vi "main.vi"() -> ()   [LabVIEW 2024]
uses:
  Controls/#typedef_program_data.ctl
  Controls/#typedef_steps.ctl
  Controls/#typedef_program_states_kawa.ctl
  Controls/#typedef_action_timer.ctl
panel:
  out "error out":errorcluster
  in  "error in (no error)":errorcluster
  in  "Cluster":T1
  in  "stop":bool
  out "Whipped Cream":bool
  out "Chocolate Syrup":bool
  out "Milk Foam":bool
  out "Steamed Milk":bool
  out "Espresso":bool
  in  "Cafe Mocha":bool
  in  "Cafe Latte":bool
  in  "Espresso Macchiato":bool
  in  "Espresso":bool
  # "Wybierz kawe:"
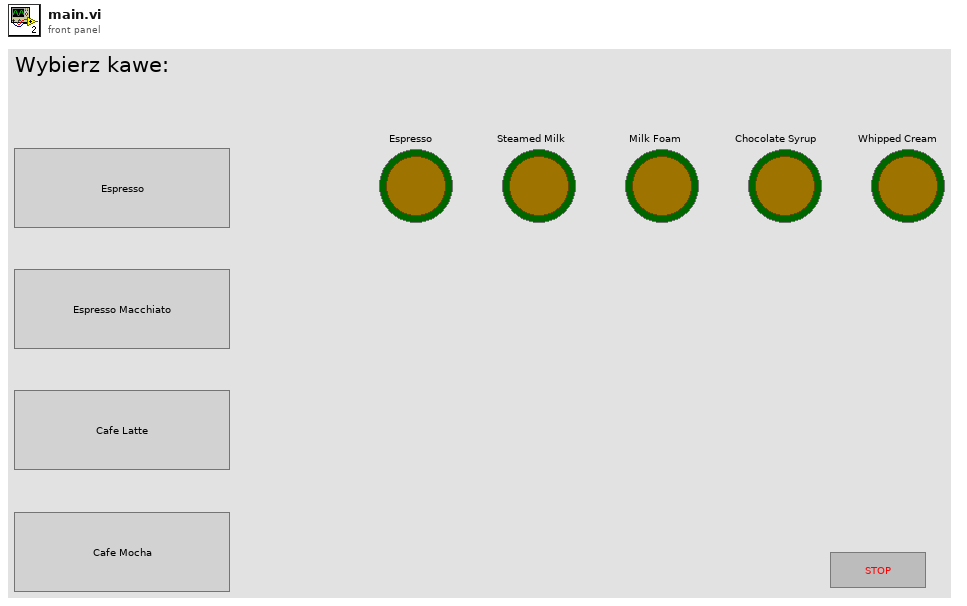
[diagram p1: front panel]
types:
  T1 = typedef "#typedef_program_data.ctl" = cluster{"Espresso":bool, "Steamed Milk":bool, "Milk Foam":bool, "Chocolate Syrup":bool, "Whipped Cream":bool, "steps":T2}
  T2 = typedef "#typedef_steps.ctl" = enum16{"start", "espresso", "chocolate syrup", "steamed milk", "milk foam", "whipped cream", "end"}
  T3 = typedef "#typedef_program_states_kawa.ctl" = enum16{"Application Error", "init", "idle", "espresso", "espresso macchiato", "caffe latte", "cafe mocha", "stop"}
  T4 = enum8{"Enabled", "Disabled", "Disabled and Grayed Out"}
  T5 = typedef "#typedef_action_timer.ctl" = enum16{"reset", "timeElapsed"}
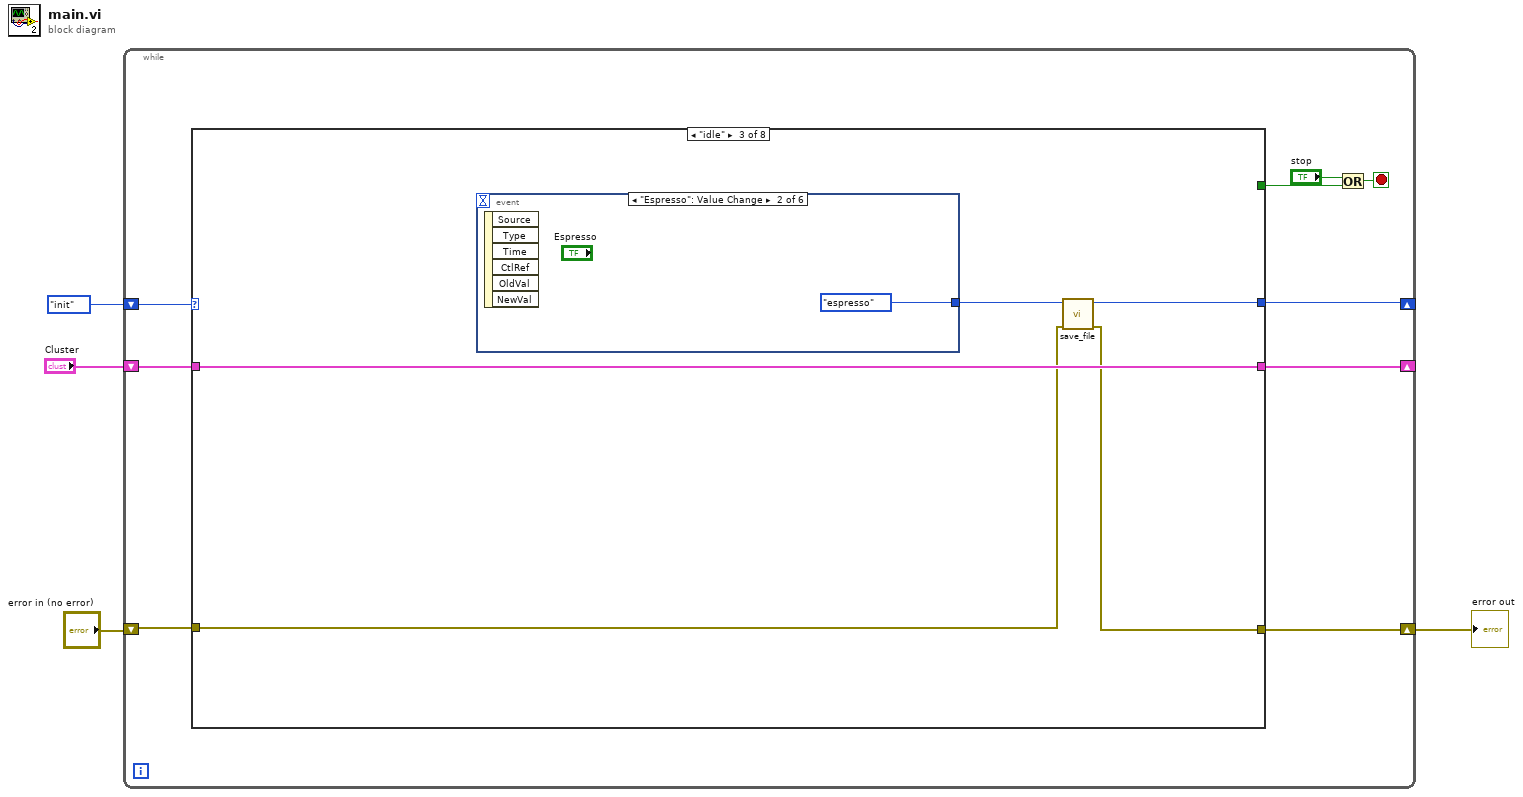
[diagram p0: block diagram]
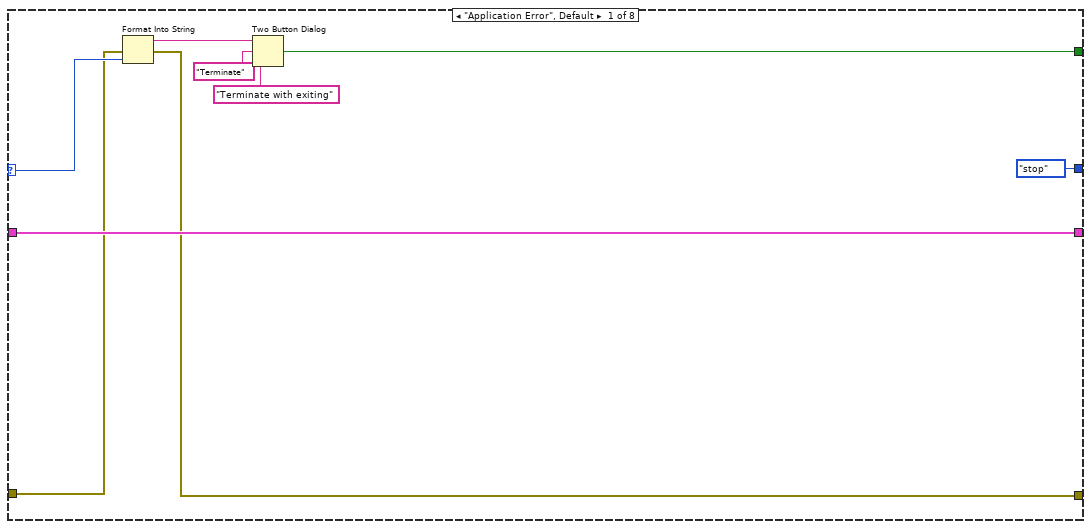
[diagram p2: hidden frame]
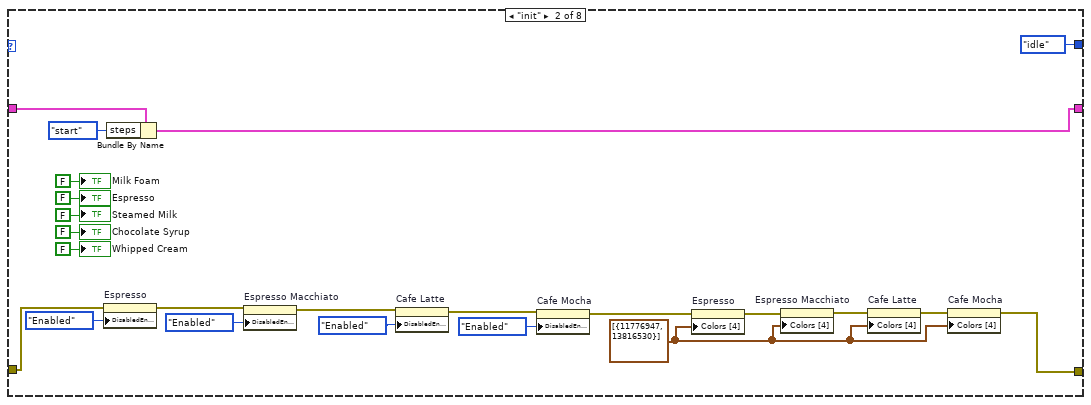
[diagram p3: hidden frame]
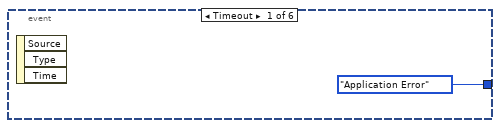
[diagram p4: hidden frame]
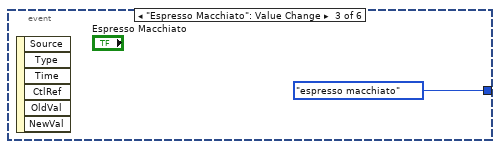
[diagram p5: hidden frame]
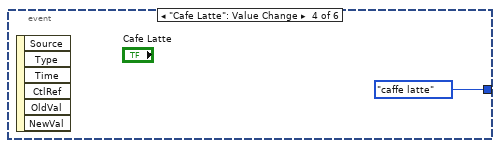
[diagram p6: hidden frame]
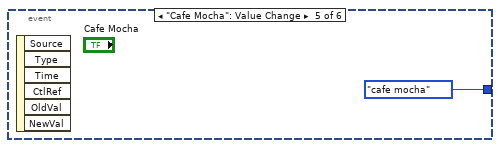
[diagram p7: hidden frame]
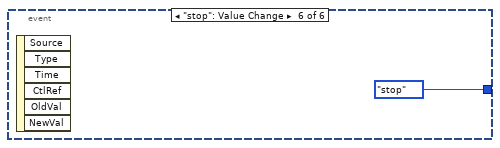
[diagram p8: hidden frame]
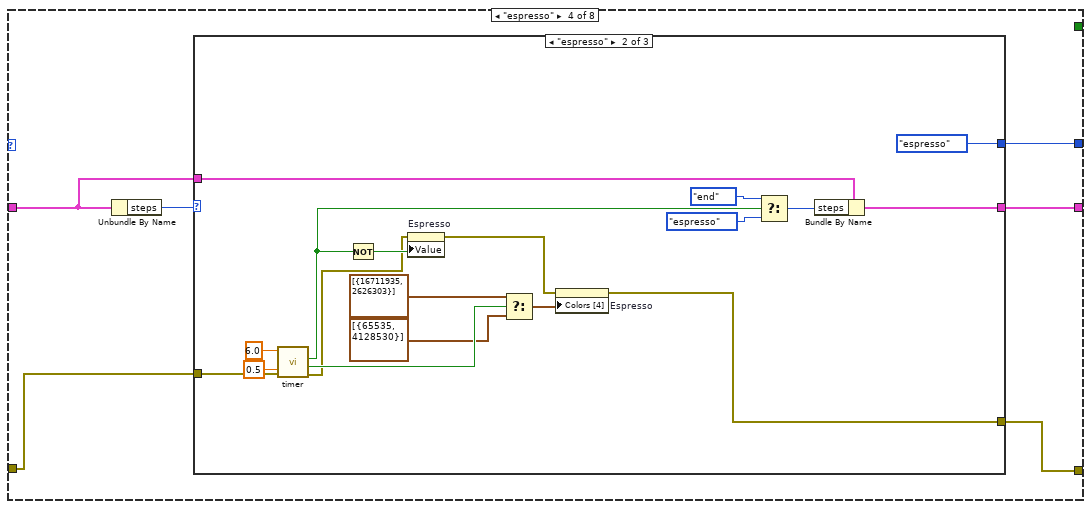
[diagram p9: hidden frame]
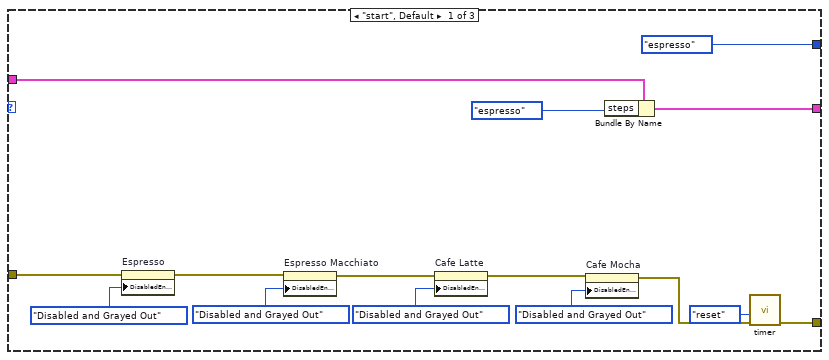
[diagram p10: hidden frame]
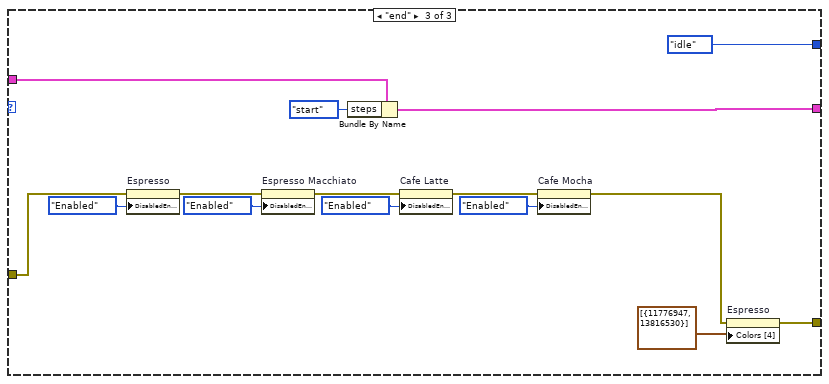
[diagram p11: hidden frame]
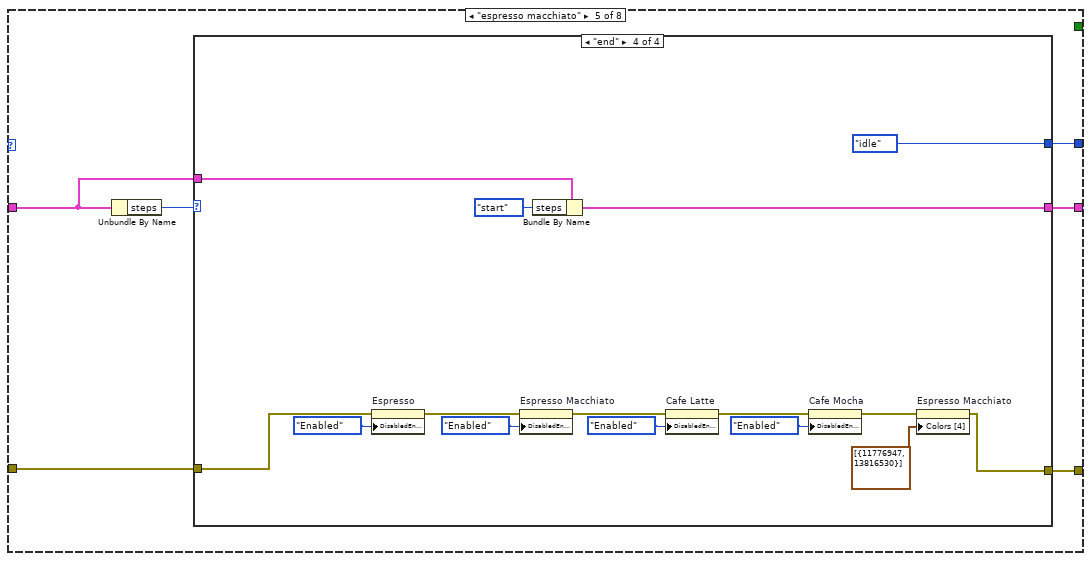
[diagram p12: hidden frame]
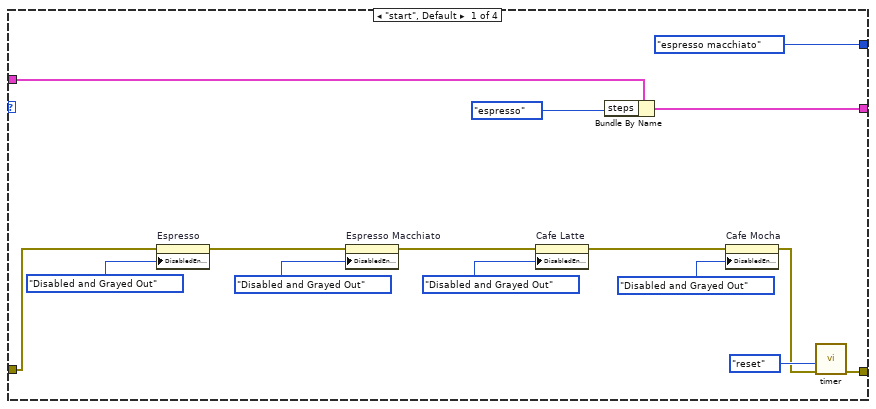
[diagram p13: hidden frame]
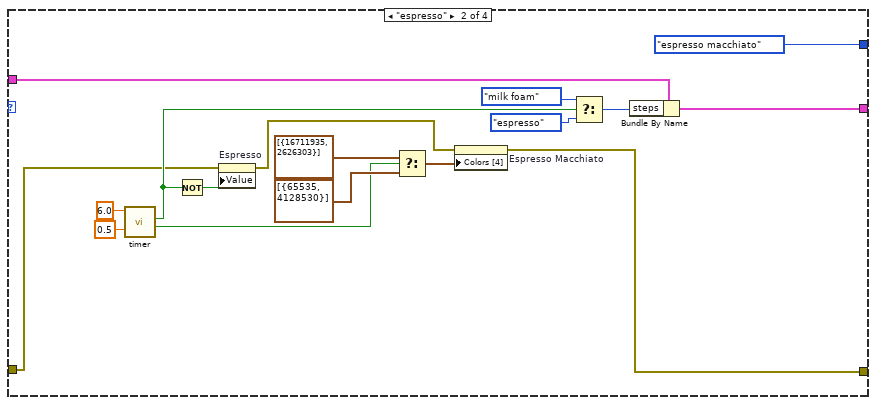
[diagram p14: hidden frame]
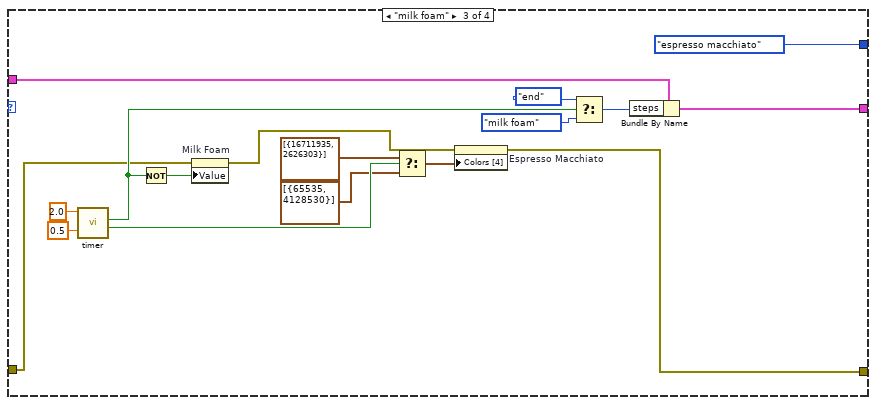
[diagram p15: hidden frame]
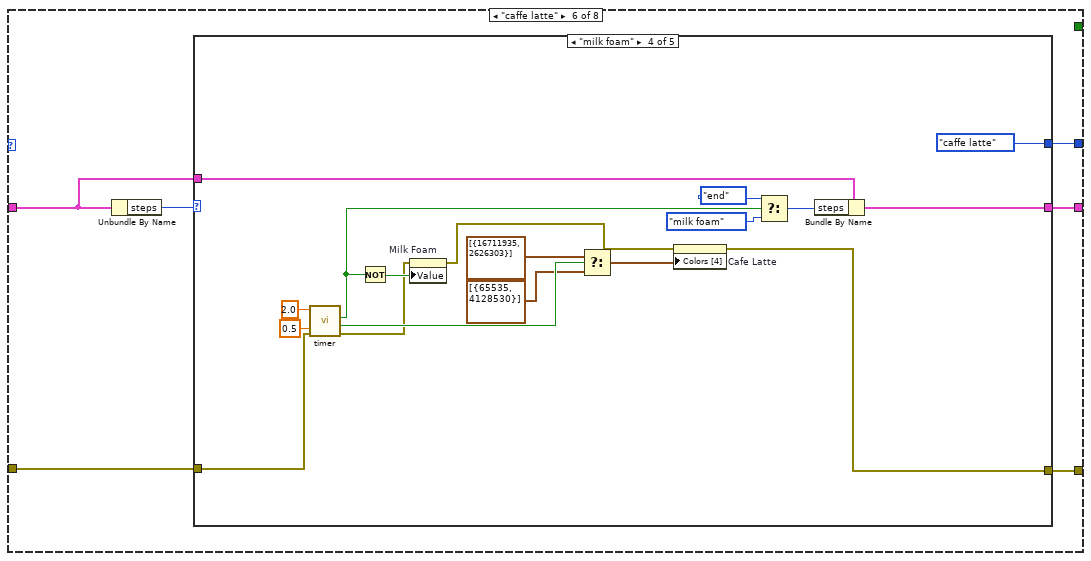
[diagram p16: hidden frame]
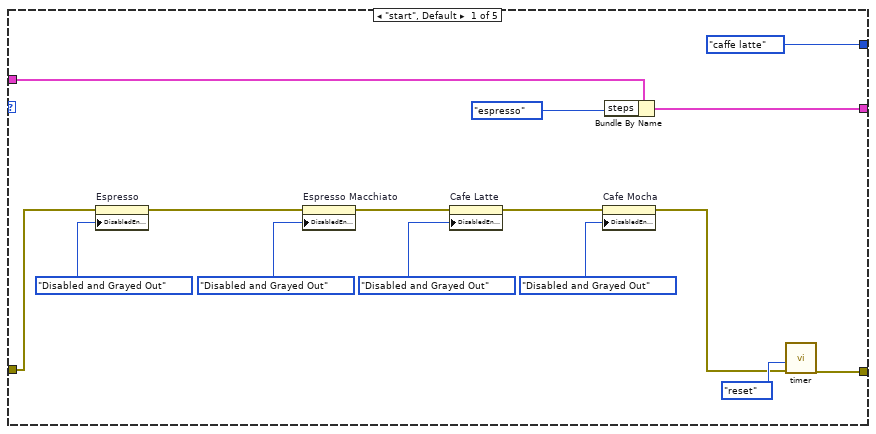
[diagram p17: hidden frame]
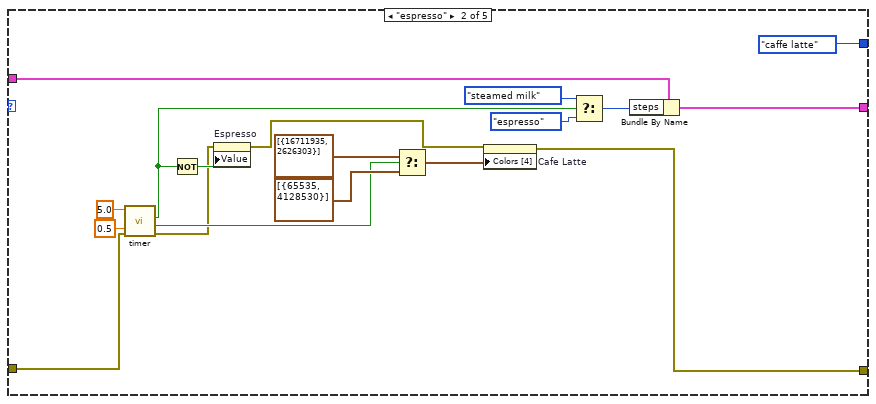
[diagram p18: hidden frame]
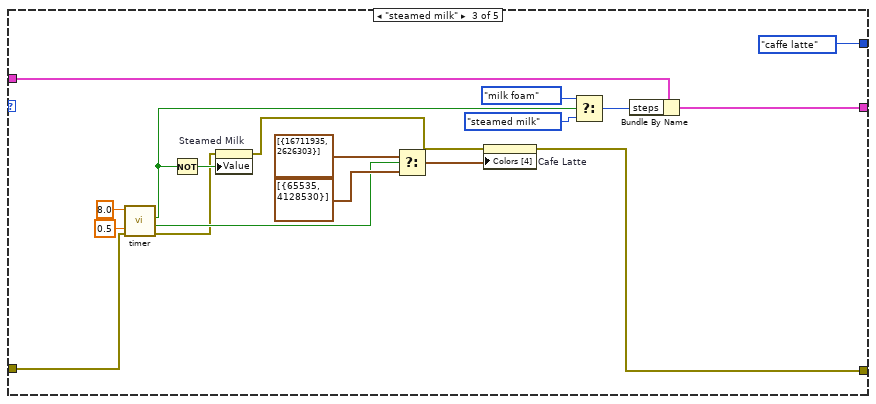
[diagram p19: hidden frame]
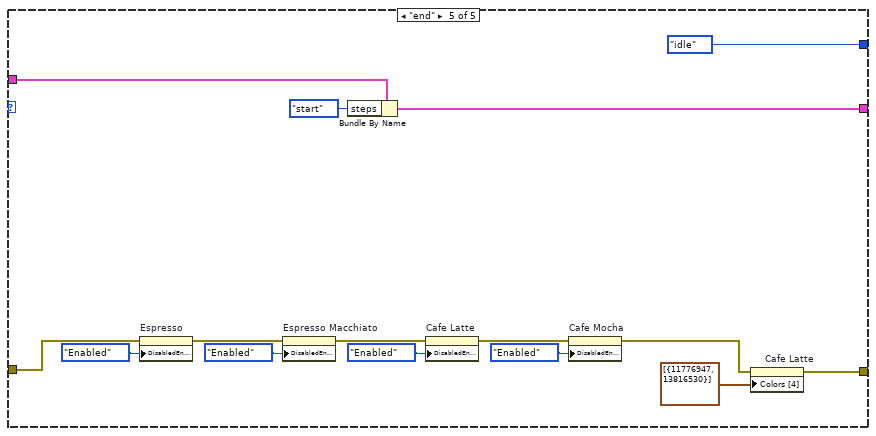
[diagram p20: hidden frame]
diagram:
  n1 = while {
    shift-right: [w11] -> _
    shift-left: #typedef_program_states_kawa."init" ("program states") -> [w13]
    shift-right: [w9] -> _
    shift-left: "Cluster" -> [w10]
    shift-right: [w5] -> w1
    shift-left: "error in (no error)" -> [w6]
    stop <- w8 stop-if-true
    n2 = case shown="\"idle\"" w13 {
      selector: w13 -> [w21 _ _ _ _ _ _ _]
      tunnel: [w17 _ _ _ _ _ _ TRUE ("T button?")] -> w12
      tunnel: [#typedef_program_states_kawa."stop" ("program states") #typedef_program_states_kawa."idle" ("program states") w48 w59 w113 w183 w273 #typedef_program_states_kawa."Application Error" ("program states")] -> w11
      tunnel: w10 -> [w16 w39 w50 w61 w115 w185 w275 w381]
      tunnel: [w16 w37 w50 w60 w114 w184 w274 w381] -> w9
      tunnel: w6 -> [w15 w31 w47 w58 w112 w182 w272 w379]
      tunnel: [w14 w23 w46 w57 w111 w181 w271 w379] -> w5
      frame "Application Error", Default {
        n3 = Format Into String(error in=w15, w21) -> (resulting string=w20:string, error out=w14:errorcluster)  [unwired: 2 in]
        n4 = Two Button Dialog(message=w20, 1:"Terminate with exiting" ("F button name (\"Cancel\")"), 2:"Terminate" ("T button name (\"OK\")")) -> (T button?=w17:bool)
      }
      frame "init" {
        w32 = cluster{u32, u32}[] [{11776947, 13816530}] ("Colors [4]")
        n5 = property on="Espresso" class="Bool"(error in=w31, "DisabledEnum"=T4."Enabled" ("Disabled")) -> (error out=w30:errorcluster)  [unwired: 1 in, 1 out]
        n6 = Bundle By Name(cluster=w39, "steps"=#typedef_steps."start") -> (w37:T1)
        n7 = property on="Espresso Macchiato" class="Bool"(error in=w30, "DisabledEnum"=T4."Enabled" ("Disabled")) -> (error out=w29:errorcluster)  [unwired: 1 in, 1 out]
        n8 = property on="Cafe Latte" class="Bool"(error in=w29, "DisabledEnum"=T4."Enabled" ("Disabled")) -> (error out=w28:errorcluster)  [unwired: 1 in, 1 out]
        n9 = property on="Cafe Mocha" class="Bool"(error in=w28, "DisabledEnum"=T4."Enabled" ("Disabled")) -> (error out=w27:errorcluster)  [unwired: 1 in, 1 out]
        n10 = property on="Espresso" class="Bool"(error in=w27, "Colors [4]"=w32) -> (error out=w26:errorcluster)  [unwired: 1 in, 1 out]
        n11 = property on="Espresso Macchiato" class="Bool"(error in=w26, "Colors [4]"=w32) -> (error out=w25:errorcluster)  [unwired: 1 in, 1 out]
        n12 = property on="Cafe Latte" class="Bool"(error in=w25, "Colors [4]"=w32) -> (error out=w24:errorcluster)  [unwired: 1 in, 1 out]
        n13 = property on="Cafe Mocha" class="Bool"(error in=w24, "Colors [4]"=w32) -> (error out=w23:errorcluster)  [unwired: 1 in, 1 out]
        "Espresso" <- FALSE ("Milk Foam")
        "Steamed Milk" <- FALSE ("Milk Foam")
        "Milk Foam" <- FALSE ("Milk Foam")
        "Chocolate Syrup" <- FALSE ("Milk Foam")
        "Whipped Cream" <- FALSE ("Milk Foam")
      }
      frame "idle" {
        n14 = event shown="[1] \"Espresso\": Value Change" {
          selector: _ -> [_ _ _ _ _ _]
          dyn-events: _ -> [_ _ _ _ _ _]
          timeout: _ -> [_ _ _ _ _ _]
          tunnel: [#typedef_program_states_kawa."Application Error" ("program states") #typedef_program_states_kawa."espresso" ("program states") #typedef_program_states_kawa."espresso macchiato" ("program states") #typedef_program_states_kawa."caffe latte" ("program states") #typedef_program_states_kawa."cafe mocha" ("program states") #typedef_program_states_kawa."stop" ("program states")] -> w49
          event Timeout {
            n15 = event-data() -> ()  [unwired: 1 in, 3 out]
          }
          event "Espresso": Value Change {
            n16 = event-data() -> ()  [unwired: 1 in, 6 out]
          }
          event "Espresso Macchiato": Value Change {
            n17 = event-data() -> ()  [unwired: 1 in, 6 out]
          }
          event "Cafe Latte": Value Change {
            n18 = event-data() -> ()  [unwired: 1 in, 6 out]
          }
          event "Cafe Mocha": Value Change {
            n19 = event-data() -> ()  [unwired: 1 in, 6 out]
          }
          event "stop": Value Change {
            n20 = event-data() -> ()  [unwired: 1 in, 6 out]
          }
        }
        n21 = call "save_file.vi"("error in (no error)"=w47, "program states  in"=w49) -> ("error out"=w46:errorcluster, "program states out"=w48:T3)  [unwired: 8 in]
      }
      frame "espresso" {
        n22 = Unbundle By Name(w61) -> ("steps"=w62:T2)
        n23 = case shown="\"espresso\"" w62 {
          tunnel: w61 -> [w77 w91 w109]
          tunnel: [w75 w92 w108] -> w60
          tunnel: [#typedef_program_states_kawa."espresso" ("program states") #typedef_program_states_kawa."espresso" ("program states") #typedef_program_states_kawa."idle" ("program states")] -> w59
          tunnel: w58 -> [w68 w81 w96]
          tunnel: [w63 w78 w101] -> w57
          frame "start", Default {
            n24 = property on="Espresso" class="Bool"(error in=w68, "DisabledEnum"=T4."Disabled and Grayed Out" ("Disabled")) -> (error out=w67:errorcluster)  [unwired: 1 in, 1 out]
            n25 = property on="Espresso Macchiato" class="Bool"(error in=w67, "DisabledEnum"=T4."Disabled and Grayed Out" ("Disabled")) -> (error out=w66:errorcluster)  [unwired: 1 in, 1 out]
            n26 = property on="Cafe Latte" class="Bool"(error in=w66, "DisabledEnum"=T4."Disabled and Grayed Out" ("Disabled")) -> (error out=w65:errorcluster)  [unwired: 1 in, 1 out]
            n27 = property on="Cafe Mocha" class="Bool"(error in=w65, "DisabledEnum"=T4."Disabled and Grayed Out" ("Disabled")) -> (error out=w64:errorcluster)  [unwired: 1 in, 1 out]
            n28 = Bundle By Name(cluster=w77, "steps"=#typedef_steps."espresso") -> (w75:T1)
            n29 = call "timer.vi"("error in (no error)"=w64, "action"=#typedef_action_timer."reset") -> ("error out"=w63:errorcluster)  [unwired: 6 in, 3 out]
          }
          frame "espresso" {
            n30 = call "timer.vi"("error in (no error)"=w81, "Time to elapse latch"=0.5, "Time to elapse (s)"=6.0) -> ("error out"=w80:errorcluster, "time elapsed latch"=w84:bool, "timeElapsed?"=w93:bool)  [unwired: 5 in, 1 out]
            n31 = Not(x=w93) -> (.not. x?=w95:bool)
            n32 = property on="Espresso" class="Bool (strict)"(error in=w80, "Value"=w95) -> (error out=w79:errorcluster)  [unwired: 1 in, 1 out]
            n33 = Select(t=cluster{u32, u32}[] [{16711935, 2626303}] ("Colors [4]"), s=w84, f=cluster{u32, u32}[] [{65535, 4128530}] ("Colors [4]")) -> (s? t:f=w86:cluster{u32, u32}[])
            n34 = property on="Espresso" class="Bool"(error in=w79, "Colors [4]"=w86) -> (error out=w78:errorcluster)  [unwired: 1 in, 1 out]
            n35 = Select(t=#typedef_steps."end" ("steps"), s=w93, f=#typedef_steps."espresso" ("steps")) -> (s? t:f=w88:T2)
            n36 = Bundle By Name(cluster=w91, "steps"=w88) -> (w92:T1)
          }
          frame "end" {
            n37 = property on="Espresso" class="Bool"(error in=w96, "DisabledEnum"=T4."Enabled" ("Disabled")) -> (error out=w97:errorcluster)  [unwired: 1 in, 1 out]
            n38 = property on="Espresso Macchiato" class="Bool"(error in=w97, "DisabledEnum"=T4."Enabled" ("Disabled")) -> (error out=w98:errorcluster)  [unwired: 1 in, 1 out]
            n39 = Bundle By Name(cluster=w109, "steps"=#typedef_steps."start") -> (w108:T1)
            n40 = property on="Cafe Latte" class="Bool"(error in=w98, "DisabledEnum"=T4."Enabled" ("Disabled")) -> (error out=w99:errorcluster)  [unwired: 1 in, 1 out]
            n41 = property on="Cafe Mocha" class="Bool"(error in=w99, "DisabledEnum"=T4."Enabled" ("Disabled")) -> (error out=w100:errorcluster)  [unwired: 1 in, 1 out]
            n42 = property on="Espresso" class="Bool"(error in=w100, "Colors [4]"=cluster{u32, u32}[] [{11776947, 13816530}]) -> (error out=w101:errorcluster)  [unwired: 1 in, 1 out]
          }
        }
      }
      frame "espresso macchiato" {
        n43 = Unbundle By Name(w115) -> ("steps"=w116:T2)
        n44 = case shown="\"end\"" w116 {
          tunnel: w115 -> [w131 w144 w162 w179]
          tunnel: [w129 w145 w163 w178] -> w114
          tunnel: [#typedef_program_states_kawa."espresso macchiato" ("program states") #typedef_program_states_kawa."espresso macchiato" ("program states") #typedef_program_states_kawa."espresso macchiato" ("program states") #typedef_program_states_kawa."idle" ("program states")] -> w113
          tunnel: w112 -> [w122 w134 w151 w171]
          tunnel: [w117 w132 w149 w166] -> w111
          frame "start", Default {
            n45 = property on="Espresso" class="Bool"(error in=w122, "DisabledEnum"=T4."Disabled and Grayed Out" ("Disabled")) -> (error out=w121:errorcluster)  [unwired: 1 in, 1 out]
            n46 = property on="Espresso Macchiato" class="Bool"(error in=w121, "DisabledEnum"=T4."Disabled and Grayed Out" ("Disabled")) -> (error out=w120:errorcluster)  [unwired: 1 in, 1 out]
            n47 = property on="Cafe Latte" class="Bool"(error in=w120, "DisabledEnum"=T4."Disabled and Grayed Out" ("Disabled")) -> (error out=w119:errorcluster)  [unwired: 1 in, 1 out]
            n48 = Bundle By Name(cluster=w131, "steps"=#typedef_steps."espresso") -> (w129:T1)
            n49 = property on="Cafe Mocha" class="Bool"(error in=w119, "DisabledEnum"=T4."Disabled and Grayed Out" ("Disabled")) -> (error out=w118:errorcluster)  [unwired: 1 in, 1 out]
            n50 = call "timer.vi"("error in (no error)"=w118, "action"=#typedef_action_timer."reset") -> ("error out"=w117:errorcluster)  [unwired: 6 in, 3 out]
          }
          frame "espresso" {
            n51 = call "timer.vi"("Time to elapse latch"=0.5, "Time to elapse (s)"=6.0) -> ("time elapsed latch"=w136:bool, "timeElapsed?"=w146:bool)  [unwired: 6 in, 2 out]
            n52 = Not(x=w146) -> (.not. x?=w148:bool)
            n53 = property on="Espresso" class="Bool (strict)"(error in=w134, "Value"=w148) -> (error out=w133:errorcluster)  [unwired: 1 in, 1 out]
            n54 = Select(t=cluster{u32, u32}[] [{16711935, 2626303}] ("Colors [4]"), s=w136, f=cluster{u32, u32}[] [{65535, 4128530}] ("Colors [4]")) -> (s? t:f=w135:cluster{u32, u32}[])
            n55 = property on="Espresso Macchiato" class="Bool"(error in=w133, "Colors [4]"=w135) -> (error out=w132:errorcluster)  [unwired: 1 in, 1 out]
            n56 = Select(t=#typedef_steps."milk foam" ("steps"), s=w146, f=#typedef_steps."espresso" ("steps")) -> (s? t:f=w141:T2)
            n57 = Bundle By Name(cluster=w144, "steps"=w141) -> (w145:T1)
          }
          frame "milk foam" {
            n58 = call "timer.vi"("Time to elapse latch"=0.5, "Time to elapse (s)"=2.0) -> ("time elapsed latch"=w156:bool, "timeElapsed?"=w164:bool)  [unwired: 6 in, 2 out]
            n59 = Not(x=w164) -> (.not. x?=w152:bool)
            n60 = property on="Milk Foam" class="Bool (strict)"(error in=w151, "Value"=w152) -> (error out=w150:errorcluster)  [unwired: 1 in, 1 out]
            n61 = Select(t=cluster{u32, u32}[] [{16711935, 2626303}] ("Colors [4]"), s=w156, f=cluster{u32, u32}[] [{65535, 4128530}] ("Colors [4]")) -> (s? t:f=w155:cluster{u32, u32}[])
            n62 = property on="Espresso Macchiato" class="Bool"(error in=w150, "Colors [4]"=w155) -> (error out=w149:errorcluster)  [unwired: 1 in, 1 out]
            n63 = Select(t=#typedef_steps."end" ("steps"), s=w164, f=#typedef_steps."milk foam" ("steps")) -> (s? t:f=w159:T2)
            n64 = Bundle By Name(cluster=w162, "steps"=w159) -> (w163:T1)
          }
          frame "end" {
            n65 = property on="Espresso" class="Bool"(error in=w171, "DisabledEnum"=T4."Enabled" ("Disabled")) -> (error out=w170:errorcluster)  [unwired: 1 in, 1 out]
            n66 = property on="Espresso Macchiato" class="Bool"(error in=w170, "DisabledEnum"=T4."Enabled" ("Disabled")) -> (error out=w169:errorcluster)  [unwired: 1 in, 1 out]
            n67 = Bundle By Name(cluster=w179, "steps"=#typedef_steps."start") -> (w178:T1)
            n68 = property on="Cafe Latte" class="Bool"(error in=w169, "DisabledEnum"=T4."Enabled" ("Disabled")) -> (error out=w168:errorcluster)  [unwired: 1 in, 1 out]
            n69 = property on="Cafe Mocha" class="Bool"(error in=w168, "DisabledEnum"=T4."Enabled" ("Disabled")) -> (error out=w167:errorcluster)  [unwired: 1 in, 1 out]
            n70 = property on="Espresso Macchiato" class="Bool"(error in=w167, "Colors [4]"=cluster{u32, u32}[] [{11776947, 13816530}]) -> (error out=w166:errorcluster)  [unwired: 1 in, 1 out]
          }
        }
      }
      frame "caffe latte" {
        n71 = Unbundle By Name(w185) -> ("steps"=w186:T2)
        n72 = case shown="\"milk foam\"" w186 {
          tunnel: w185 -> [w201 w215 w234 w252 w269]
          tunnel: [w199 w216 w235 w253 w268] -> w184
          tunnel: [#typedef_program_states_kawa."caffe latte" ("program states") #typedef_program_states_kawa."caffe latte" ("program states") #typedef_program_states_kawa."caffe latte" ("program states") #typedef_program_states_kawa."caffe latte" ("program states") #typedef_program_states_kawa."idle" ("program states")] -> w183
          tunnel: w182 -> [w187 w202 w220 w238 w261]
          tunnel: [w192 w204 w222 w240 w256] -> w181
          frame "start", Default {
            n73 = property on="Espresso" class="Bool"(error in=w187, "DisabledEnum"=T4."Disabled and Grayed Out" ("Disabled")) -> (error out=w188:errorcluster)  [unwired: 1 in, 1 out]
            n74 = property on="Espresso Macchiato" class="Bool"(error in=w188, "DisabledEnum"=T4."Disabled and Grayed Out" ("Disabled")) -> (error out=w189:errorcluster)  [unwired: 1 in, 1 out]
            n75 = property on="Cafe Latte" class="Bool"(error in=w189, "DisabledEnum"=T4."Disabled and Grayed Out" ("Disabled")) -> (error out=w190:errorcluster)  [unwired: 1 in, 1 out]
            n76 = property on="Cafe Mocha" class="Bool"(error in=w190, "DisabledEnum"=T4."Disabled and Grayed Out" ("Disabled")) -> (error out=w191:errorcluster)  [unwired: 1 in, 1 out]
            n77 = Bundle By Name(cluster=w201, "steps"=#typedef_steps."espresso") -> (w199:T1)
            n78 = call "timer.vi"("error in (no error)"=w191, "action"=#typedef_action_timer."reset") -> ("error out"=w192:errorcluster)  [unwired: 6 in, 3 out]
          }
          frame "espresso" {
            n79 = call "timer.vi"("error in (no error)"=w202, "Time to elapse latch"=0.5, "Time to elapse (s)"=5.0) -> ("error out"=w203:errorcluster, "time elapsed latch"=w207:bool, "timeElapsed?"=w217:bool)  [unwired: 5 in, 1 out]
            n80 = Not(x=w217) -> (.not. x?=w219:bool)
            n81 = property on="Espresso" class="Bool (strict)"(error in=w203, "Value"=w219) -> (error out=w205:errorcluster)  [unwired: 1 in, 1 out]
            n82 = Select(t=cluster{u32, u32}[] [{16711935, 2626303}] ("Colors [4]"), s=w207, f=cluster{u32, u32}[] [{65535, 4128530}] ("Colors [4]")) -> (s? t:f=w206:cluster{u32, u32}[])
            n83 = property on="Cafe Latte" class="Bool"(error in=w205, "Colors [4]"=w206) -> (error out=w204:errorcluster)  [unwired: 1 in, 1 out]
            n84 = Select(t=#typedef_steps."steamed milk" ("steps"), s=w217, f=#typedef_steps."espresso" ("steps")) -> (s? t:f=w212:T2)
            n85 = Bundle By Name(cluster=w215, "steps"=w212) -> (w216:T1)
          }
          frame "steamed milk" {
            n86 = call "timer.vi"("error in (no error)"=w220, "Time to elapse latch"=0.5, "Time to elapse (s)"=8.0) -> ("error out"=w221:errorcluster, "time elapsed latch"=w226:bool, "timeElapsed?"=w236:bool)  [unwired: 5 in, 1 out]
            n87 = Not(x=w236) -> (.not. x?=w224:bool)
            n88 = property on="Steamed Milk" class="Bool (strict)"(error in=w221, "Value"=w224) -> (error out=w223:errorcluster)  [unwired: 1 in, 1 out]
            n89 = Select(t=cluster{u32, u32}[] [{16711935, 2626303}] ("Colors [4]"), s=w226, f=cluster{u32, u32}[] [{65535, 4128530}] ("Colors [4]")) -> (s? t:f=w225:cluster{u32, u32}[])
            n90 = property on="Cafe Latte" class="Bool"(error in=w223, "Colors [4]"=w225) -> (error out=w222:errorcluster)  [unwired: 1 in, 1 out]
            n91 = Select(t=#typedef_steps."milk foam" ("steps"), s=w236, f=#typedef_steps."steamed milk" ("steps")) -> (s? t:f=w231:T2)
            n92 = Bundle By Name(cluster=w234, "steps"=w231) -> (w235:T1)
          }
          frame "milk foam" {
            n93 = call "timer.vi"("error in (no error)"=w238, "Time to elapse latch"=0.5, "Time to elapse (s)"=2.0) -> ("error out"=w239:errorcluster, "time elapsed latch"=w246:bool, "timeElapsed?"=w254:bool)  [unwired: 5 in, 1 out]
            n94 = Not(x=w254) -> (.not. x?=w243:bool)
            n95 = property on="Milk Foam" class="Bool (strict)"(error in=w239, "Value"=w243) -> (error out=w241:errorcluster)  [unwired: 1 in, 1 out]
            n96 = Select(t=cluster{u32, u32}[] [{16711935, 2626303}] ("Colors [4]"), s=w246, f=cluster{u32, u32}[] [{65535, 4128530}] ("Colors [4]")) -> (s? t:f=w242:cluster{u32, u32}[])
            n97 = property on="Cafe Latte" class="Bool"(error in=w241, "Colors [4]"=w242) -> (error out=w240:errorcluster)  [unwired: 1 in, 1 out]
            n98 = Select(t=#typedef_steps."end" ("steps"), s=w254, f=#typedef_steps."milk foam" ("steps")) -> (s? t:f=w249:T2)
            n99 = Bundle By Name(cluster=w252, "steps"=w249) -> (w253:T1)
          }
          frame "end" {
            n100 = property on="Espresso" class="Bool"(error in=w261, "DisabledEnum"=T4."Enabled" ("Disabled")) -> (error out=w260:errorcluster)  [unwired: 1 in, 1 out]
            n101 = property on="Espresso Macchiato" class="Bool"(error in=w260, "DisabledEnum"=T4."Enabled" ("Disabled")) -> (error out=w259:errorcluster)  [unwired: 1 in, 1 out]
            n102 = Bundle By Name(cluster=w269, "steps"=#typedef_steps."start") -> (w268:T1)
            n103 = property on="Cafe Latte" class="Bool"(error in=w259, "DisabledEnum"=T4."Enabled" ("Disabled")) -> (error out=w258:errorcluster)  [unwired: 1 in, 1 out]
            n104 = property on="Cafe Mocha" class="Bool"(error in=w258, "DisabledEnum"=T4."Enabled" ("Disabled")) -> (error out=w257:errorcluster)  [unwired: 1 in, 1 out]
            n105 = property on="Cafe Latte" class="Bool"(error in=w257, "Colors [4]"=cluster{u32, u32}[] [{11776947, 13816530}]) -> (error out=w256:errorcluster)  [unwired: 1 in, 1 out]
          }
        }
      }
      frame "cafe mocha" {
        n106 = Unbundle By Name(w275) -> ("steps"=w276:T2)
        n107 = case shown="\"espresso\"" w276 {
          tunnel: w275 -> [w291 w305 w324 w342 w360 w377]
          tunnel: [w289 w306 w325 w343 w361 w376] -> w274
          tunnel: [#typedef_program_states_kawa."cafe mocha" ("program states") #typedef_program_states_kawa."cafe mocha" ("program states") #typedef_program_states_kawa."cafe mocha" ("program states") #typedef_program_states_kawa."cafe mocha" ("program states") #typedef_program_states_kawa."cafe mocha" ("program states") #typedef_program_states_kawa."idle" ("program states")] -> w273
          tunnel: w272 -> [w277 w294 w313 w330 w347 w364]
          tunnel: [w282 w292 w310 w328 w346 w365] -> w271
          frame "start", Default {
            n108 = property on="Espresso" class="Bool"(error in=w277, "DisabledEnum"=T4."Disabled and Grayed Out" ("Disabled")) -> (error out=w278:errorcluster)  [unwired: 1 in, 1 out]
            n109 = property on="Espresso Macchiato" class="Bool"(error in=w278, "DisabledEnum"=T4."Disabled and Grayed Out" ("Disabled")) -> (error out=w279:errorcluster)  [unwired: 1 in, 1 out]
            n110 = property on="Cafe Latte" class="Bool"(error in=w279, "DisabledEnum"=T4."Disabled and Grayed Out" ("Disabled")) -> (error out=w280:errorcluster)  [unwired: 1 in, 1 out]
            n111 = Bundle By Name(cluster=w291, "steps"=#typedef_steps."espresso") -> (w289:T1)
            n112 = property on="Cafe Mocha" class="Bool"(error in=w280, "DisabledEnum"=T4."Disabled and Grayed Out" ("Disabled")) -> (error out=w281:errorcluster)  [unwired: 1 in, 1 out]
            n113 = call "timer.vi"("error in (no error)"=w281, "action"=#typedef_action_timer."reset") -> ("error out"=w282:errorcluster)  [unwired: 6 in, 3 out]
          }
          frame "espresso" {
            n114 = call "timer.vi"("error in (no error)"=w294, "Time to elapse latch"=0.5, "Time to elapse (s)"=5.0) -> ("error out"=w295:errorcluster, "time elapsed latch"=w297:bool, "timeElapsed?"=w307:bool)  [unwired: 5 in, 1 out]
            n115 = Not(x=w307) -> (.not. x?=w309:bool)
            n116 = property on="Espresso" class="Bool (strict)"(error in=w295, "Value"=w309) -> (error out=w293:errorcluster)  [unwired: 1 in, 1 out]
            n117 = Select(t=cluster{u32, u32}[] [{16711935, 2626303}] ("Colors [4]"), s=w297, f=cluster{u32, u32}[] [{65535, 4128530}] ("Colors [4]")) -> (s? t:f=w296:cluster{u32, u32}[])
            n118 = property on="Cafe Mocha" class="Bool"(error in=w293, "Colors [4]"=w296) -> (error out=w292:errorcluster)  [unwired: 1 in, 1 out]
            n119 = Select(t=#typedef_steps."chocolate syrup" ("steps"), s=w307, f=#typedef_steps."espresso" ("steps")) -> (s? t:f=w302:T2)
            n120 = Bundle By Name(cluster=w305, "steps"=w302) -> (w306:T1)
          }
          frame "chocolate syrup" {
            n121 = call "timer.vi"("error in (no error)"=w313, "Time to elapse latch"=0.5, "Time to elapse (s)"=2.0) -> ("error out"=w312:errorcluster, "time elapsed latch"=w316:bool, "timeElapsed?"=w326:bool)  [unwired: 5 in, 1 out]
            n122 = Not(x=w326) -> (.not. x?=w314:bool)
            n123 = property on="Chocolate Syrup" class="Bool (strict)"(error in=w312, "Value"=w314) -> (error out=w311:errorcluster)  [unwired: 1 in, 1 out]
            n124 = Select(t=cluster{u32, u32}[] [{16711935, 2626303}] ("Colors [4]"), s=w316, f=cluster{u32, u32}[] [{65535, 4128530}] ("Colors [4]")) -> (s? t:f=w315:cluster{u32, u32}[])
            n125 = property on="Cafe Mocha" class="Bool"(error in=w311, "Colors [4]"=w315) -> (error out=w310:errorcluster)  [unwired: 1 in, 1 out]
            n126 = Select(t=#typedef_steps."steamed milk" ("steps"), s=w326, f=#typedef_steps."chocolate syrup" ("steps")) -> (s? t:f=w321:T2)
            n127 = Bundle By Name(cluster=w324, "steps"=w321) -> (w325:T1)
          }
          frame "steamed milk" {
            n128 = call "timer.vi"("error in (no error)"=w330, "Time to elapse latch"=0.5, "Time to elapse (s)"=2.0) -> ("error out"=w331:errorcluster, "time elapsed latch"=w334:bool, "timeElapsed?"=w344:bool)  [unwired: 5 in, 1 out]
            n129 = Not(x=w344) -> (.not. x?=w333:bool)
            n130 = property on="Steamed Milk" class="Bool (strict)"(error in=w331, "Value"=w333) -> (error out=w329:errorcluster)  [unwired: 1 in, 1 out]
            n131 = Select(t=cluster{u32, u32}[] [{16711935, 2626303}] ("Colors [4]"), s=w334, f=cluster{u32, u32}[] [{65535, 4128530}] ("Colors [4]")) -> (s? t:f=w332:cluster{u32, u32}[])
            n132 = property on="Cafe Mocha" class="Bool"(error in=w329, "Colors [4]"=w332) -> (error out=w328:errorcluster)  [unwired: 1 in, 1 out]
            n133 = Select(t=#typedef_steps."whipped cream" ("steps"), s=w344, f=#typedef_steps."steamed milk" ("steps")) -> (s? t:f=w339:T2)
            n134 = Bundle By Name(cluster=w342, "steps"=w339) -> (w343:T1)
          }
          frame "whipped cream" {
            n135 = call "timer.vi"("error in (no error)"=w347, "Time to elapse latch"=0.5, "Time to elapse (s)"=2.0) -> ("error out"=w348:errorcluster, "time elapsed latch"=w352:bool, "timeElapsed?"=w362:bool)  [unwired: 5 in, 1 out]
            n136 = Not(x=w362) -> (.not. x?=w351:bool)
            n137 = property on="Whipped Cream" class="Bool (strict)"(error in=w348, "Value"=w351) -> (error out=w349:errorcluster)  [unwired: 1 in, 1 out]
            n138 = Select(t=cluster{u32, u32}[] [{16711935, 2626303}] ("Colors [4]"), s=w352, f=cluster{u32, u32}[] [{65535, 4128530}] ("Colors [4]")) -> (s? t:f=w350:cluster{u32, u32}[])
            n139 = property on="Cafe Mocha" class="Bool"(error in=w349, "Colors [4]"=w350) -> (error out=w346:errorcluster)  [unwired: 1 in, 1 out]
            n140 = Select(t=#typedef_steps."end" ("steps"), s=w362, f=#typedef_steps."whipped cream" ("steps")) -> (s? t:f=w357:T2)
            n141 = Bundle By Name(cluster=w360, "steps"=w357) -> (w361:T1)
          }
          frame "end" {
            n142 = property on="Espresso" class="Bool"(error in=w364, "DisabledEnum"=T4."Enabled" ("Disabled")) -> (error out=w369:errorcluster)  [unwired: 1 in, 1 out]
            n143 = property on="Espresso Macchiato" class="Bool"(error in=w369, "DisabledEnum"=T4."Enabled" ("Disabled")) -> (error out=w368:errorcluster)  [unwired: 1 in, 1 out]
            n144 = Bundle By Name(cluster=w377, "steps"=#typedef_steps."start") -> (w376:T1)
            n145 = property on="Cafe Latte" class="Bool"(error in=w368, "DisabledEnum"=T4."Enabled" ("Disabled")) -> (error out=w367:errorcluster)  [unwired: 1 in, 1 out]
            n146 = property on="Cafe Mocha" class="Bool"(error in=w367, "DisabledEnum"=T4."Enabled" ("Disabled")) -> (error out=w366:errorcluster)  [unwired: 1 in, 1 out]
            n147 = property on="Cafe Mocha" class="Bool"(error in=w366, "Colors [4]"=cluster{u32, u32}[] [{11776947, 13816530}]) -> (error out=w365:errorcluster)  [unwired: 1 in, 1 out]
          }
        }
      }
      frame "stop" {
      }
    }
    n148 = Or(x="stop", y=w12) -> (x .or. y?=w8:bool)
  }
  "error out" <- w1
